vi "ENTRADA-SALIDA CAN.vi"(5 "ID":string, 6 "Data":string, 7 "interface":refnum<k21>) -> (0 "Identifier":u32 format="%x", 1 "Payload":u8[](array[numeric]), 2 "ID String":string, 3 "Timestamp":timestamp, 4 "Data Type":T1 items=["CAN Data"=0, "CAN Remote"=1, "CAN Bus Error"=2, "CAN 2.0 Data"=8, "CAN FD Data"=16, "CAN FD+BRS Data"=24, "J1939 Data"=192, "Delay"=224, "Log Trigger"=225, "Start Trigger"=226])   [LabVIEW 2022 SP3]
uses:
  <vilib>/xnet/xnet.llb/XNET Frame Type CAN.ctl
  <vilib>/xnet/xnet.llb/XNET Frame CAN.ctl
panel:
  out "cluster":T3 {"data[0]"."payload" format="%x"; "data[0]"."timestamp" format="%<%.7X\n%x>T"; "data[0]"."type" items=["CAN Data"=0, "CAN Remote"=1, "CAN Bus Error"=2, "CAN 2.0 Data"=8, "CAN FD Data"=16, "CAN FD+BRS Data"=24, "J1939 Data"=192, "Delay"=224, "Log Trigger"=225, "Start Trigger"=226]; "data[0]"."identifier" format="%x"; "data[1]"."payload" format="%x"; "data[1]"."timestamp" format="%<%.7X\n%x>T"; "data[1]"."type" items=["CAN Data"=0, "CAN Remote"=1, "CAN Bus Error"=2, "CAN 2.0 Data"=8, "CAN FD Data"=16, "CAN FD+BRS Data"=24, "J1939 Data"=192, "Delay"=224, "Log Trigger"=225, "Start Trigger"=226]; "data[1]"."identifier" format="%x"; "data[2]"."payload" format="%x"; "data[2]"."timestamp" format="%<%.7X\n%x>T"; "data[2]"."type" items=["CAN Data"=0, "CAN Remote"=1, "CAN Bus Error"=2, "CAN 2.0 Data"=8, "CAN FD Data"=16, "CAN FD+BRS Data"=24, "J1939 Data"=192, "Delay"=224, "Log Trigger"=225, "Start Trigger"=226]; "data[2]"."identifier" format="%x"; "data[3]"."payload" format="%x"; "data[3]"."timestamp" format="%<%.7X\n%x>T"; "data[3]"."type" items=["CAN Data"=0, "CAN Remote"=1, "CAN Bus Error"=2, "CAN 2.0 Data"=8, "CAN FD Data"=16, "CAN FD+BRS Data"=24, "J1939 Data"=192, "Delay"=224, "Log Trigger"=225, "Start Trigger"=226]; "data[3]"."identifier" format="%x"; "data[4]"."payload" format="%x"; "data[4]"."timestamp" format="%<%.7X\n%x>T"; "data[4]"."type" items=["CAN Data"=0, "CAN Remote"=1, "CAN Bus Error"=2, "CAN 2.0 Data"=8, "CAN FD Data"=16, "CAN FD+BRS Data"=24, "J1939 Data"=192, "Delay"=224, "Log Trigger"=225, "Start Trigger"=226]; "data[4]"."identifier" format="%x"; "data[5]"."payload" format="%x"; "data[5]"."timestamp" format="%<%.7X\n%x>T"; "data[5]"."type" items=["CAN Data"=0, "CAN Remote"=1, "CAN Bus Error"=2, "CAN 2.0 Data"=8, "CAN FD Data"=16, "CAN FD+BRS Data"=24, "J1939 Data"=192, "Delay"=224, "Log Trigger"=225, "Start Trigger"=226]; "data[5]"."identifier" format="%x"; "data[6]"."payload" format="%x"; "data[6]"."timestamp" format="%<%.7X\n%x>T"; "data[6]"."type" items=["CAN Data"=0, "CAN Remote"=1, "CAN Bus Error"=2, "CAN 2.0 Data"=8, "CAN FD Data"=16, "CAN FD+BRS Data"=24, "J1939 Data"=192, "Delay"=224, "Log Trigger"=225, "Start Trigger"=226]; "data[6]"."identifier" format="%x"; "data[7]"."payload" format="%x"; "data[7]"."timestamp" format="%<%.7X\n%x>T"; "data[7]"."type" items=["CAN Data"=0, "CAN Remote"=1, "CAN Bus Error"=2, "CAN 2.0 Data"=8, "CAN FD Data"=16, "CAN FD+BRS Data"=24, "J1939 Data"=192, "Delay"=224, "Log Trigger"=225, "Start Trigger"=226]; "data[7]"."identifier" format="%x"; "data[8]"."payload" format="%x"; "data[8]"."timestamp" format="%<%.7X\n%x>T"; "data[8]"."type" items=["CAN Data"=0, "CAN Remote"=1, "CAN Bus Error"=2, "CAN 2.0 Data"=8, "CAN FD Data"=16, "CAN FD+BRS Data"=24, "J1939 Data"=192, "Delay"=224, "Log Trigger"=225, "Start Trigger"=226]; "data[8]"."identifier" format="%x"}
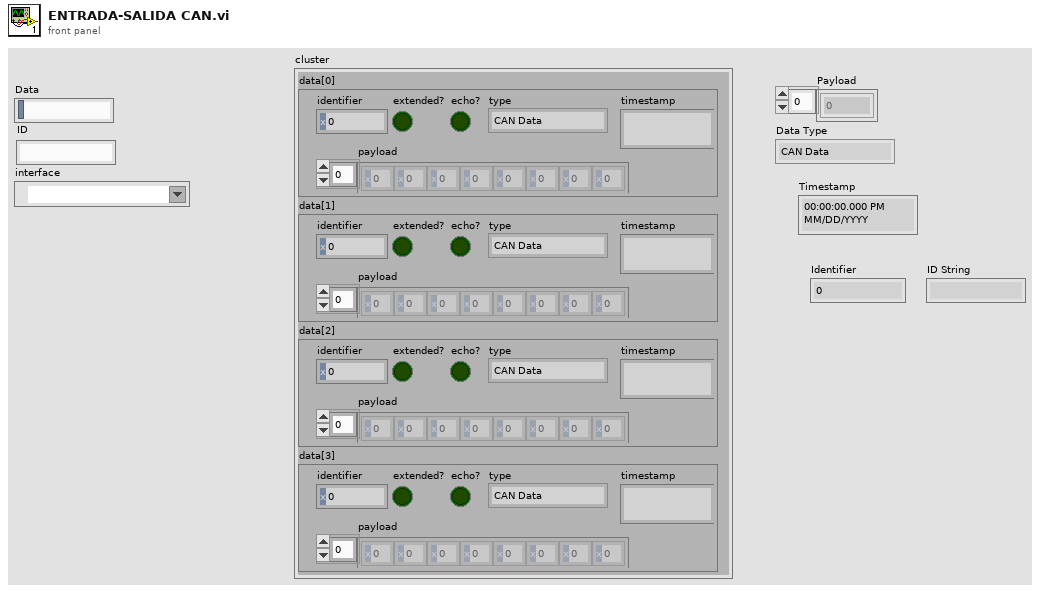
[diagram p1: front panel]
types:
  T1 = typedef "XNET Frame Type CAN.ctl" = u8
  T2 = typedef "XNET Frame CAN.ctl" = cluster{"timestamp":timestamp, "payload":u8[], "identifier":u32, "type":T1, "extended?":bool, "echo?":bool}
  T3 = cluster{"data[0]":T2, "data[1]":T2, "data[2]":T2, "data[3]":T2, "data[4]":T2, "data[5]":T2, "data[6]":T2, "data[7]":T2, "data[8]":T2}
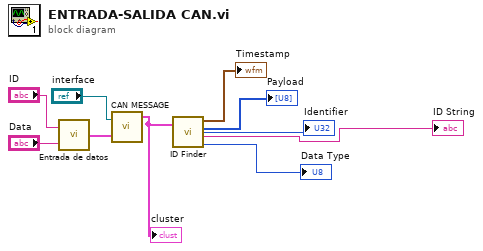
[diagram p0: block diagram]
diagram:
  n1 = call "Entrada de datos.vi"("string"="Data", "ID"="ID") -> ("CAN frame"=w7:T2)
  n2 = call "CAN MESSAGE.vi"("interface"="interface", "CAN frame"=w7) -> ("cluster"=w6:T3)  [unwired: 1 in, 1 out]
  "cluster" <- w6
  n3 = call "ID Finder.vi"("cluster"=w6) -> ("Data Type"=→"Data Type":T1, "ID STRING"=→"ID String":string, "Payload"=→"Payload":u8[], "Timestamp"=→"Timestamp":timestamp, "Identifier"=→"Identifier":u32)  [unwired: 1 in]
